vi "Create Pattern Script(Addr).vi"(8 "error in (no error)":errorcluster, 10 "Addr":u16, 11 "SPI 4W Pattern Creator in":refnum<class "SPI 4W Pattern Creator.lvclass">) -> (0 "error out":errorcluster, 2 "String":string, 3 "SPI 4W Pattern Creator out":refnum<class "SPI 4W Pattern Creator.lvclass">)   [LabVIEW 2018, in "SPI 4W Pattern Creator.lvlib" / "SPI 4W Pattern Creator.lvclass"]
uses:
  SPI 4W Pattern Creator.lvclass
  Interfaces/Protocol Interface.lvlibp/Interfaces/Protocol Interface/Pin State.ctl
  Interfaces/Protocol Interface.lvlibp/Interfaces/Protocol Interface/Protocol Interface.lvclass
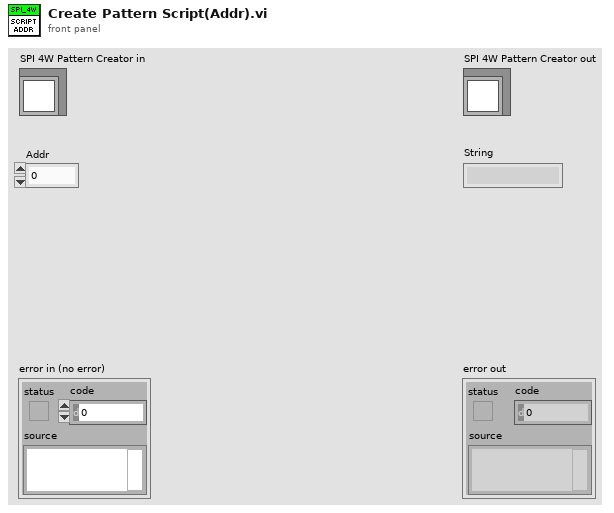
[diagram p1: front panel]
types:
  T1 = typedef "Protocol Interface.lvlibp/Protocol Interface.lvclass/Pin State.ctl" = enum16{"0", "1", "L", "H", "X", "V", "D", "M"}
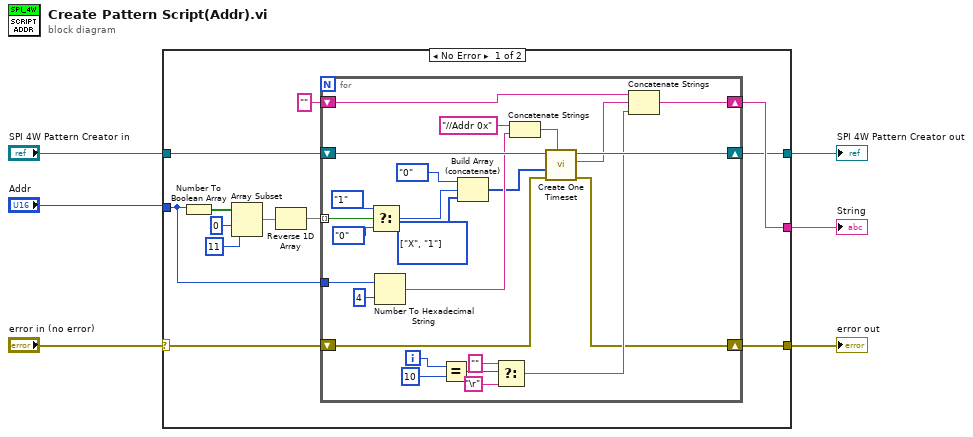
[diagram p0: block diagram]
diagram:
  n1 = case shown="No Error" "error in (no error)" {
    selector: "error in (no error)" -> [w11 w45]
    tunnel: "SPI 4W Pattern Creator in" -> [w12 w44]
    tunnel: "Addr" -> [w13 _]
    tunnel: [w9 _] -> w3
    tunnel: [w8 w44] -> w1
    tunnel: [w7 w45] -> w2
    frame No Error {
      n2 = Number To Boolean Array(number=w13) -> (Boolean array=w18:bool[])
      n3 = Array Subset(array=w18, index=0, length=11) -> (w15:bool[])
      n4 = Reverse 1D Array(array=w15) -> (reversed array=w14:bool[])
      n5 = for {
        tunnel: w14 -> [w41] mode=indexing
        tunnel: w13 -> [w38]
        shift-right: [w33] -> w8
        shift-left: w12 -> [w43]
        shift-right: [w23] -> w7
        shift-left: w11 -> [w42]
        shift-right: [w31] -> w9
        shift-left: "" -> [w30]
        i -> [w29]
        w19 = T1[] [enum."X", enum."1"] items=["0", "1", "L", "H", "X", "V", "D", "M"] ("PinStates")
        n6 = Select(t=Pin_State."1" ("PinState"), s=w41, f=Pin_State."0") -> (s? t:f=w22:T1)
        n7 = Number To Hexadecimal String(1:i16 4 ("width (-)"), 2:w38) -> (0:w34:string)
        n8 = Equal?(x=w29, y=10) -> (x = y?=w27:bool)
        n9 = Build Array (concatenate)(Pin_State."0" ("element"), w22, w19) -> (w20:T1[])
        n10 = Select(t="", s=w27, f="\r") -> (s? t:f=w24:string)
        n11 = Concatenate Strings("//Addr 0x" ("string"), w34) -> (w36:string)
        n12 = call-dynamic "Create One Timeset.vi"("Notes"=w36, "error in (no error)"=w42, "PinStates"=w20, "SPI 4W Pattern Creator in"=w43) -> ("error out"=w23:errorcluster, "String  out"=w32:string, "SPI 4W Pattern Creator out"=w33:refnum<class "SPI 4W Pattern Creator.lvclass">)  [unwired: 5 in]
        n13 = Concatenate Strings(w30, w32, w24) -> (w31:string)
      }
    }
    frame Error {
    }
  }
  "error out" <- w2
  "SPI 4W Pattern Creator out" <- w1
  "String" <- w3
